vi "get parameter min and max.vi"(8 "error in (no error)":errorcluster, 9 "parameter name":string, 10 "limit values":string[][](array[string])) -> (0 "error out":errorcluster, 1 "min":dbl, 2 "max":dbl)   [LabVIEW 2018]
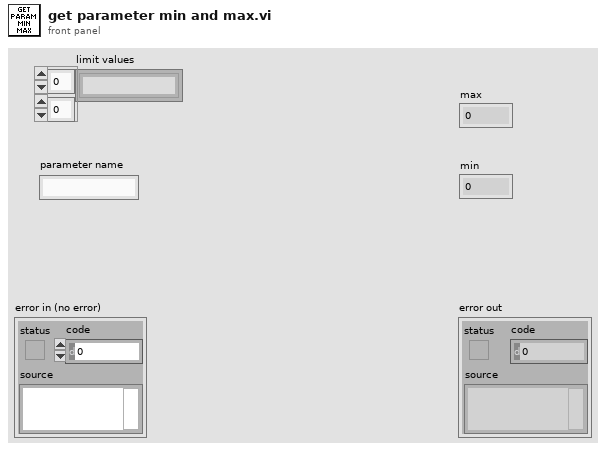
[diagram p1: front panel]
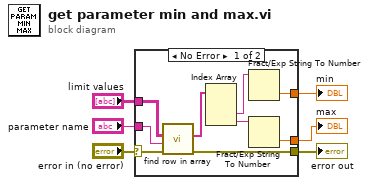
[diagram p0: block diagram]
diagram:
  n1 = case shown="No Error" "error in (no error)" {
    selector: "error in (no error)" -> [w8 w16]
    tunnel: [w13 w16] -> w5
    tunnel: [w15 _] -> w4
    tunnel: [w14 _] -> w3
    tunnel: "parameter name" -> [w9 _]
    tunnel: "limit values" -> [w7 _]
    frame No Error {
      n2 = call "find row in array.vi"("error in (no error)"=w8, "parameter name"=w9, "limit values"=w7) -> ("error out"=w13:errorcluster, "row"=w12:string[])  [unwired: 7 in]
      n3 = Index Array(array=w12) -> (element #2=w11:string, element #3=w10:string)  [unwired: 3 in, 1 out]
      n4 = Fract/Exp String To Number(string=w11) -> (number=w15:dbl)  [unwired: 3 in, 1 out]
      n5 = Fract/Exp String To Number(string=w10) -> (number=w14:dbl)  [unwired: 3 in, 1 out]
    }
    frame Error {
    }
  }
  "error out" <- w5
  "max" <- w3
  "min" <- w4
